vi "Direct Call.vi"(7 "Actor in":refnum<class "Actor.lvclass">, 9 "Error":errorcluster, 10 "Actor":refnum<class "Actor.lvclass">) -> (0 "Error out":errorcluster, 5 "Actor out":refnum<class "Actor.lvclass">)   [LabVIEW 2025, in "jettl.lvlib" / "Terminate Msg.lvlib"]
uses:
  Terminate Msg.lvlib
  Actor/Actor/Actor.lvclass
  Terminate Msg/Terminate Msg.lvclass
  C:/git/jettl/src/jettl/jettl/Msg/Msg.lvclass
  Actor/Actor.lvlib
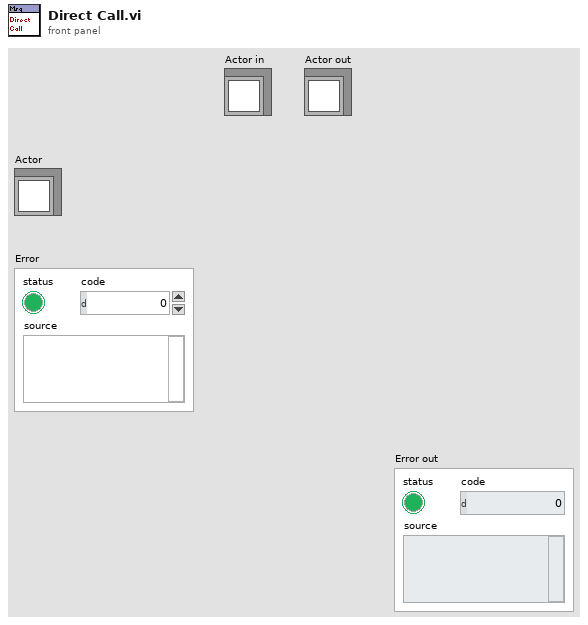
[diagram p1: front panel]
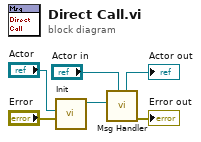
[diagram p0: block diagram]
diagram:
  n1 = call "Init.vi"("Error"="Error", "Actor"="Actor") -> ("Terminate Msg out"=w3:refnum<class "Terminate Msg.lvclass">)  [unwired: 9 in]
  n2 = call "Msg Handler.vi"("Actor in"="Actor in", "Msg"=w3) -> ("Error out"=→"Error out":errorcluster, "Actor out"=→"Actor out":refnum<class "Actor.lvclass">)  [unwired: 8 in]
